vi "FIB beam blank.vi"(2 "ActiveX Container":refnum<k7>(container), 3 "Beam blanked":bool, 5 "lines":tag="FIB/port0/line0") -> (0 "error out":errorcluster)   [LabVIEW 2018]
uses:
  <vilib>/DAQmx/write.llb/DAQmx Write (Digital Bool 1Line 1Point).vi
  <vilib>/DAQmx/create/channels.llb/DAQmx Create Channel (DO-Digital Output).vi
  <vilib>/DAQmx/miscellaneous.llb/DAQmx Fill In Error Info.vi
panel:
  in  "Machine Type":u8(ring) items=["Feiss", "NVision", "Jeiss"]
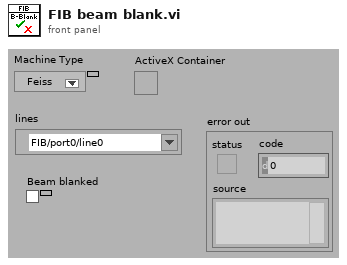
[diagram p1: front panel]
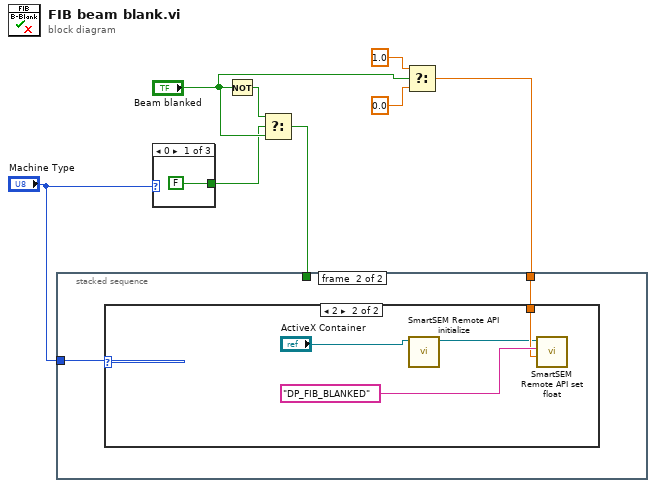
[diagram p0: block diagram]
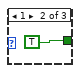
[diagram p2: hidden frame]
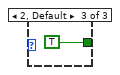
[diagram p3: hidden frame]
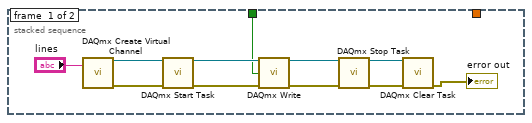
[diagram p4: hidden frame]
diagram:
  n1 = case shown="0" "Machine Type" {
    tunnel: [FALSE ("Low blanked") TRUE ("Low blanked") TRUE ("Low blanked")] -> w1
    frame 0 {
    }
    frame 1 {
    }
    frame 2, Default {
    }
  }
  n2 = Not(x="Beam blanked") -> (.not. x?=w7:bool)
  n3 = Select(t=w7, s=w1, f="Beam blanked") -> (s? t:f=w8:bool)
  n4 = Select(t=sgl 1.0, s="Beam blanked", f=sgl 0.0) -> (s? t:f=w3:sgl)
  n5 = stacked-sequence {
    tunnel: w8 -> [w15 _]
    tunnel: w3 -> [_ w24]
    tunnel: "Machine Type" -> [_ w23]
    frame #0 {
      n6 = call-poly <vilib>:"DAQmx Create Virtual Channel.vi"("lines"="lines") -> ("task out"=w22:refnum<k21>, "error out"=w21:errorcluster)  [unwired: 13 in]
      n7 = call <vilib>:"DAQmx Start Task.vi"("task/channels in"=w22, "error in"=w21) -> ("task out"=w20:refnum<k21>, "error out"=w19:errorcluster)  [unwired: 12 in]
      n8 = call-poly <vilib>:"DAQmx Write.vi"("task/channels in"=w20, "data"=w15, "error in"=w19) -> ("task out"=w18:refnum<k21>, "error out"=w17:errorcluster)  [unwired: 10 in, 1 out]
      n9 = call <vilib>:"DAQmx Stop Task.vi"("task/channels in"=w18, "error in"=w17) -> ("task out"=w13:refnum<k21>, "error out"=w14:errorcluster)  [unwired: 12 in]
      n10 = call <vilib>:"DAQmx Clear Task.vi"("task in"=w13, "error in"=w14) -> ("error out"=→"error out":errorcluster)  [unwired: 13 in]
    }
    frame #1 {
      n11 = case shown="2" w23 {
        tunnel: w24 -> [_ w27]
        frame 0, Default {
        }
        frame 2 {
          n12 = call "SmartSEM Remote API initialize.vi"("ActiveX Container"="ActiveX Container") -> ("reference out"=w25:refnum<k7>)  [unwired: 9 in, 1 out]
          n13 = call "SmartSEM Remote API set float.vi"("vValue"=w27, "lpszParam"="DP_FIB_BLANKED", "ActiveX Container"=w25) -> ()  [unwired: 7 in, 2 out]
        }
      }
    }
  }
